vi "Write Bottom.vi"(8 "error in (no error)":errorcluster, 10 "Bottom":i16, 11 "Image Assertion in":refnum<class "Image Assertion.lvclass">) -> (0 "error out":errorcluster, 3 "Image Assertion out":refnum<class "Image Assertion.lvclass">)   [LabVIEW 2020, in "MacroAssert.lvlib" / "Image Assertion.lvclass"]
uses:
  Image Assertion.lvclass
  Image Assertion.lvclass/Image Assertion.ctl
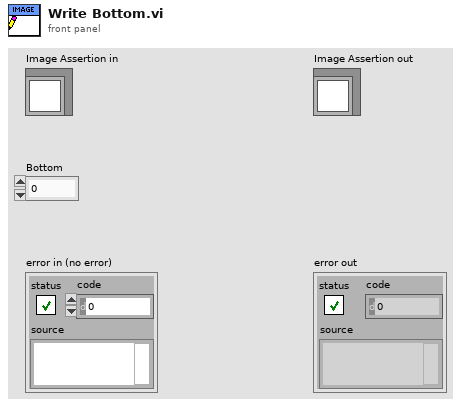
[diagram p1: front panel]
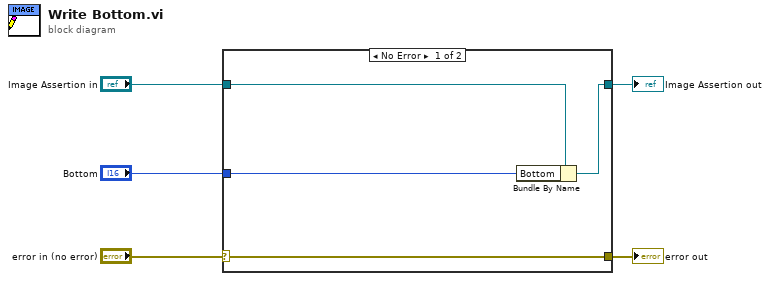
[diagram p0: block diagram]
diagram:
  n1 = case shown="No Error" "error in (no error)" {
    selector: "error in (no error)" -> [w9 w10]
    tunnel: [w9 w10] -> w4
    tunnel: [w7 w11] -> w2
    tunnel: "Image Assertion in" -> [w8 w11]
    tunnel: "Bottom" -> [w6 _]
    frame No Error {
      n2 = Bundle By Name(cluster=w8, "Bottom"=w6) -> (w7:refnum<class "Image Assertion.lvclass">)
    }
    frame Error {
    }
  }
  "error out" <- w4
  "Image Assertion out" <- w2
